vi "XML Get.vi"(8 "error in (no error)":errorcluster, 9 "Data Type":string, 10 "Parameter":string, 11 "XML String in":string) -> (0 "error out":errorcluster, 3 "Value":string)   [LabVIEW 2021, in "BS120x Driver.lvlib" / "ENET_BS1200.lvclass"]
uses:
  ENET_BS1200.lvclass
  <vilib>/xml/Close Reference(Node).vi
  <resource>/objmgr/DOMUserDefRef.rc
  <vilib>/xml/NI_XML.lvlib
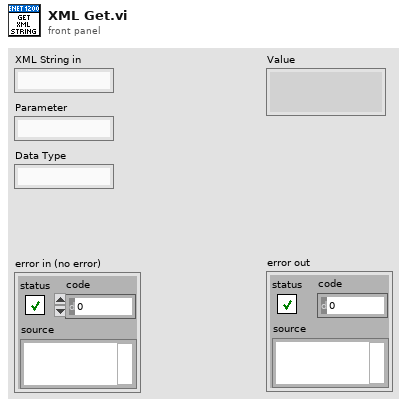
[diagram p1: front panel]
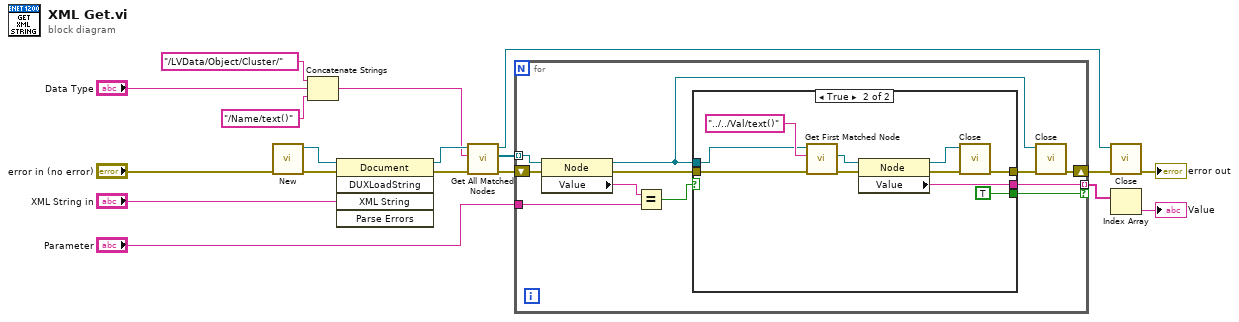
[diagram p0: block diagram]
diagram:
  n1 = call <vilib>:"New.vi"("error in (no error)"="error in (no error)") -> ("error out"=w17:errorcluster, "DOM document out"=w18:refnum<k20>)  [unwired: 7 in]
  n2 = Concatenate Strings("/LVData/Object/Cluster/" ("XPath expression"), "Data Type", "/Name/text()" ("string")) -> (w11:string)
  n3 = invoke class="Document" method="DUXLoadString"(reference=w18, error in=w17, "XML String"="XML String in") -> (reference out=w14:refnum<k20>, error out=w15:errorcluster)  [unwired: 2 in, 3 out]
  n4 = call <vilib>:"Get All Matched Nodes.vi"("error in (no error)"=w15, "XPath expression"=w11, "node in"=w14) -> ("error out"=w13:errorcluster, "node result array"=w12:refnum<k20>[], "node out"=w4:refnum<k20>)  [unwired: 6 in]
  n5 = for {
    shift-right: [w24] -> w3
    shift-left: w13 -> [w29]
    tunnel: w12 -> [w28] mode=indexing
    tunnel: "Parameter" -> [w23]
    tunnel: [w20] -> w2 mode=indexing if=w19
    n6 = property class="Node"(reference=w28, error in=w29) -> (reference out=w26:refnum<k20>, error out=w27:errorcluster, "Value"=w22:string)
    n7 = Equal?(x=w22, y=w23) -> (x = y?=w21:bool)
    n8 = case shown="True" w21 {
      tunnel: w26 -> [_ w34]
      tunnel: w27 -> [w30 w38]
      tunnel: [w30 w33] -> w25
      tunnel: [_ w32] -> w20
      tunnel: [_ TRUE] -> w19
      frame False {
      }
      frame True {
        n9 = call <vilib>:"Get First Matched Node.vi"("error in (no error)"=w38, "XPath expression"="../../Val/text()", "node in"=w34) -> ("error out"=w36:errorcluster, "node result"=w35:refnum<k20>)  [unwired: 6 in, 1 out]
        n10 = property class="Node"(reference=w35, error in=w36) -> (reference out=w39:refnum<k20>, error out=w40:errorcluster, "Value"=w32:string)
        n11 = call-poly <vilib>:"Close.vi"("error in (no error)"=w40, "node"=w39) -> ("error out"=w33:errorcluster)  [unwired: 7 in]
      }
    }
    n12 = call-poly <vilib>:"Close.vi"("error in (no error)"=w25, "node"=w26) -> ("error out"=w24:errorcluster)  [unwired: 7 in]
  }
  n13 = call-poly <vilib>:"Close.vi"("error in (no error)"=w3, "node"=w4) -> ("error out"=→"error out":errorcluster)  [unwired: 7 in]
  n14 = Index Array(array=w2) -> (element=→"Value":string)  [unwired: 1 in]
